vi "NI6602.CreateServices.vi"(0 "i ref in":refnum<vi>, 2 "name":string, 3 "Address":string[](array[string]), 5 "error in (no error)":errorcluster) -> (14 "i ref out":refnum<vi>, 19 "error out":errorcluster)   [LabVIEW 2014, in "NI6602.lvlib"]
doc: "Creates all services.\n\nLicense Agreement for this software:\n\nCopyright (C)\nGesellschaft für Schwerionenforschung, GSI\nPlanckstr. 1\n64291 Darmstadt\nGermany\n\nContact: D.Beck@gsi.de \n\nThis program is free software; you can redistribute it and/or modify it under the terms of the \nGNU General Public License as published by the Free Software Foundation; either version 2 of \nthe license, or (at your option) any later version.\n\nThis program is distributed in the hope that it will be useful, but WITHOUT ANY WARRANTY; \nwithout even the implied warranty of MERCHANTABILITY or FITNESS FOR A PARTICULAR PURPOSE. See the GNU General License for more details (http://www.gnu.org).\n\nGesellschaft für Schwerionenforschung, GSI\nPlanckstr. 1, 64291 Darmstadt, Germany\nFor all questions and ideas contact: M.Richter@gsi.de, H.Brand@gsi.de or D.Beck@gsi.de.\nLast update: 16-JUN-2004"
uses:
  NI6602.lvlib
  CSlibraries-extern/DimLVEvent/LVDimInterface/LVDimInterface.lvlib
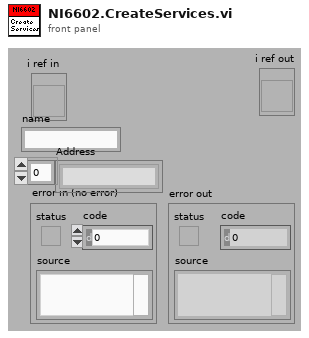
[diagram p1: front panel]
types:
  T1 = typedef "NI6602.lvlib/NI6602.i attribute.ctl" = cluster{"CounterDAQ Channels":cluster{"task":refnum<k21>, "Channel Name":string}[], "RateServiceIDs":i32[], "Running?":bool, "IntegralServiceIDs":i32[], "ThresholdID":i32, "Threshold":dbl, "IntegralValues":dbl[], "Stopped?":bool}
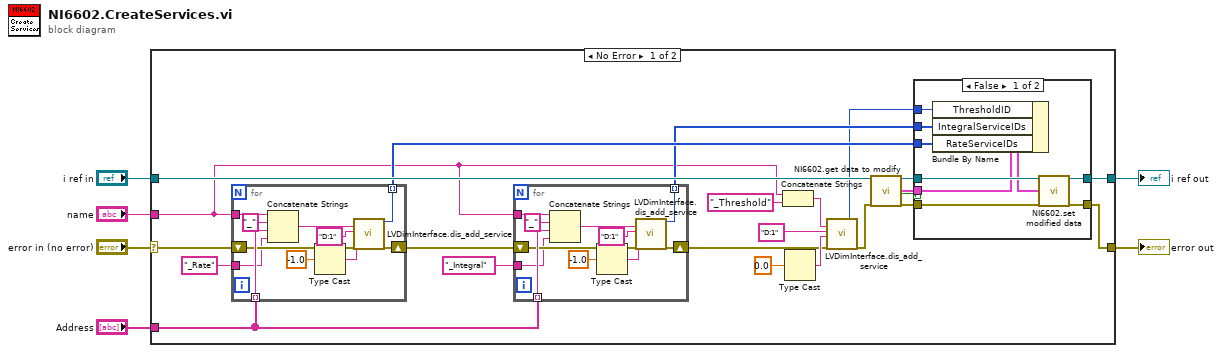
[diagram p0: block diagram]
diagram:
  n1 = case shown="No Error" "error in (no error)" {
    selector: "error in (no error)" -> [w25 w64]
    tunnel: [w23 w63] -> w6
    tunnel: [w22 w64] -> w5
    tunnel: "i ref in" -> [w24 w63]
    tunnel: "name" -> [w9 _]
    tunnel: "Address" -> [w18 _]
    frame No Error {
      n2 = for {
        tunnel: w9 -> [w61]
        tunnel: w18 -> [w59] mode=indexing
        shift-right: [w57] -> w19
        shift-left: w25 -> [w58]
        tunnel: [w53] -> w21 mode=indexing
        tunnel: "_Rate" ("string") -> [w52]
        n3 = Concatenate Strings(w61, "_" ("string"), w59, w52) -> (w62:string)
        n4 = Type Cast(x=-1.0) -> (*(type *) &x=w56:string)  [unwired: 1 in]
        n5 = call "LVDimInterface.dis_add_service.vi"("serviceName"=w62, "typeDescriptor"="D:1", "data"=w56, "error in (no error)"=w58) -> ("my_serviceID"=w53:i32, "error out"=w57:errorcluster)  [unwired: 14 in]
      }
      n6 = for {
        tunnel: w9 -> [w39]
        tunnel: w18 -> [w37] mode=indexing
        shift-right: [w35] -> w11
        shift-left: w19 -> [w36]
        tunnel: [w31] -> w16 mode=indexing
        tunnel: "_Integral" ("string") -> [w30]
        n7 = Concatenate Strings(w39, "_" ("string"), w37, w30) -> (w40:string)
        n8 = Type Cast(x=-1.0) -> (*(type *) &x=w34:string)  [unwired: 1 in]
        n9 = call "LVDimInterface.dis_add_service.vi"("serviceName"=w40, "typeDescriptor"="D:1", "data"=w34, "error in (no error)"=w36) -> ("my_serviceID"=w31:i32, "error out"=w35:errorcluster)  [unwired: 14 in]
      }
      n10 = Concatenate Strings(w9, "_Threshold" ("string")) -> (w10:string)
      n11 = Type Cast(x=0.0) -> (*(type *) &x=w15:string)  [unwired: 1 in]
      n12 = call "LVDimInterface.dis_add_service.vi"("serviceName"=w10, "typeDescriptor"="D:1", "data"=w15, "error in (no error)"=w11) -> ("my_serviceID"=w8:i32, "error out"=w7:errorcluster)  [unwired: 14 in]
      n13 = call "NI6602.get data to modify.vi"("i ref in"=w24, "error in (no error)"=w7) -> ("i ref out"=w26:refnum<vi>, "i attribute"=w29:T1, "timed out"=w28:bool, "error out"=w27:errorcluster)  [unwired: 14 in]
      n14 = case shown="False" w28 {
        tunnel: w26 -> [w49 w51]
        tunnel: [w48 w51] -> w23
        tunnel: w27 -> [w47 w50]
        tunnel: [w46 w50] -> w22
        tunnel: w29 -> [w45 _]
        tunnel: w21 -> [w43 _]
        tunnel: w16 -> [w42 _]
        tunnel: w8 -> [w41 _]
        frame False {
          n15 = Bundle By Name(cluster=w45, "ThresholdID"=w41, "IntegralServiceIDs"=w42, "RateServiceIDs"=w43) -> (w44:T1)
          n16 = call "NI6602.set modified data.vi"("i ref in"=w49, "i attribute"=w44, "error in (no error)"=w47) -> ("i ref out"=w48:refnum<vi>, "error out"=w46:errorcluster)  [unwired: 15 in]
        }
        frame True {
        }
      }
    }
    frame Error {
    }
  }
  "i ref out" <- w6
  "error out" <- w5
